vi "Write Formatters.vi"(8 "error in (no error)":errorcluster, 10 "Formatters":refnum<class "Formatter Config.lvclass">[](array[class]), 11 "OnTheFlyReport Config in":refnum<class "OnTheFlyReport Config.lvclass">) -> (0 "error out":errorcluster, 3 "OnTheFlyReport Config out":refnum<class "OnTheFlyReport Config.lvclass">)   [LabVIEW 2015, in "OnTheFlyReport Config.lvclass"]
uses:
  OnTheFlyReport Config.lvclass
  Report Formatters/Base Class/Config/Formatter Config.lvclass
  OnTheFlyReport Config.lvclass/OnTheFlyReport Config.ctl
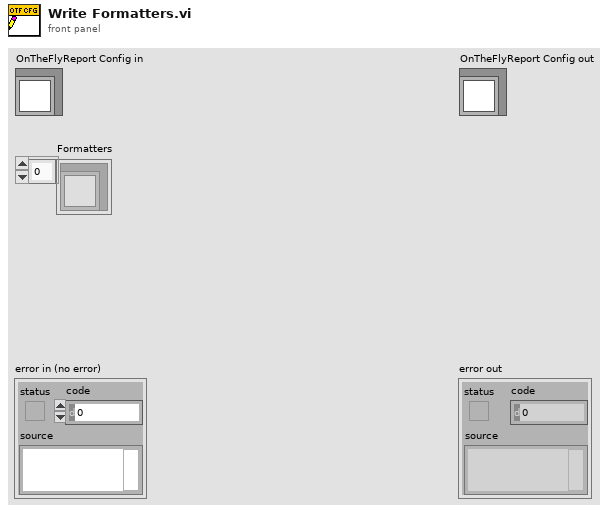
[diagram p1: front panel]
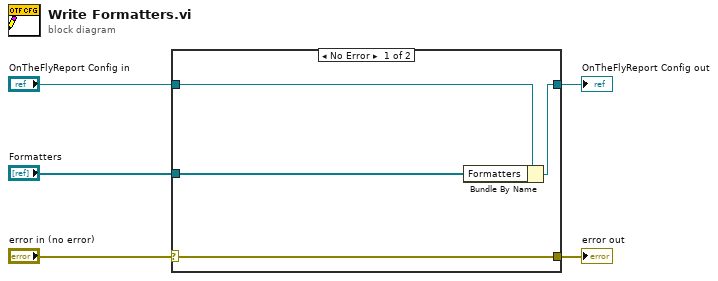
[diagram p0: block diagram]
diagram:
  n1 = case shown="No Error" "error in (no error)" {
    selector: "error in (no error)" -> [w9 w10]
    tunnel: [w9 w10] -> w4
    tunnel: [w7 w11] -> w2
    tunnel: "OnTheFlyReport Config in" -> [w8 w11]
    tunnel: "Formatters" -> [w6 _]
    frame No Error {
      n2 = Bundle By Name(cluster=w8, "Formatters"=w6) -> (w7:refnum<class "OnTheFlyReport Config.lvclass">)
    }
    frame Error {
    }
  }
  "error out" <- w4
  "OnTheFlyReport Config out" <- w2
